vi "1.vi"   [LabVIEW 2017]
types:
  T1 = enum16{"open", "replace", "create", "open or create", "replace or create", "replace or create with confirmation"}
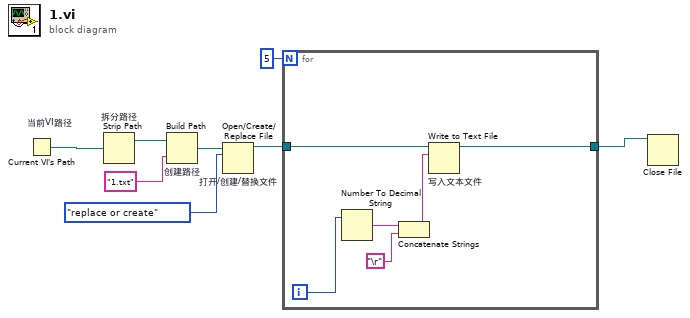
[diagram p0: block diagram]
diagram:
  n1 = Current VI's Path "当前VI路径"() -> (path=w8:path)
  n2 = Strip Path "拆分路径"(path=w8) -> (stripped path=w7:path)  [unwired: 1 out]
  n3 = Build Path "创建路径"(base path=w7, name or relative path="1.txt" ("名称或相对路径")) -> (appended path=w5:path)
  n4 = Open/Create/Replace File "打开/创建/替换文件"(file path (use dialog)=w5, operation (0:open)=T1."replace or create" ("操作(0:open)")) -> (refnum out=w2:refnum<file>)  [unwired: 4 in, 2 out]
  n5 = for {
    N: 5 -> [_]
    tunnel: w2 -> [w14]
    tunnel: [w9] -> w1
    i -> [w13]
    n6 = Number To Decimal String(number=w13) -> (decimal integer string=w12:string)  [unwired: 1 in]
    n7 = Concatenate Strings(w12, "\r") -> (w10:string)
    n8 = Write to Text File "写入文本文件"(file (use dialog)=w14, text=w10) -> (refnum out=w9:refnum<file>)  [unwired: 2 in, 2 out]
  }
  n9 = Close File(refnum=w1) -> ()  [unwired: 1 in, 2 out]
